vi "Clean Up.vi"(8 "error in (no error)":errorcluster, 11 "1553 Component in":refnum<class "1553 Component.lvclass">) -> (0 "error out":errorcluster)   [LabVIEW 2020, in "BCI-1553 API.lvlib" / "1553 Component.lvclass"]
doc: "Performs clean-up on the component. This will generally prepare the component in the 1553 Session to a known state and make it ready to accept a new configuration."
uses:
  1553 Component.lvclass
  1553 Component.lvclass/1553 Component.ctl
  Dependencies/FPGA Interface/FPGA Interface.lvclass
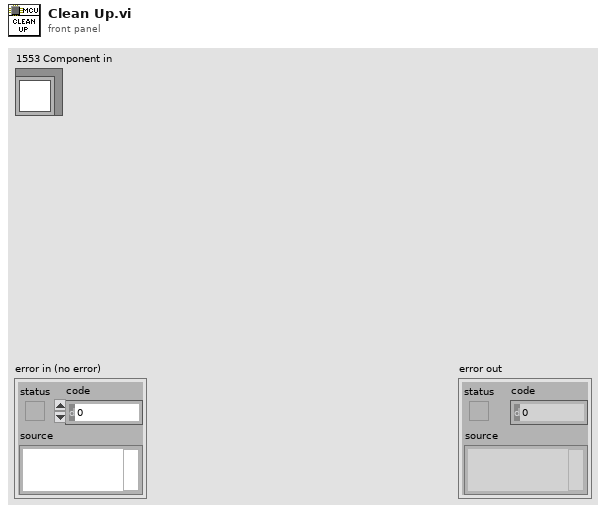
[diagram p1: front panel]
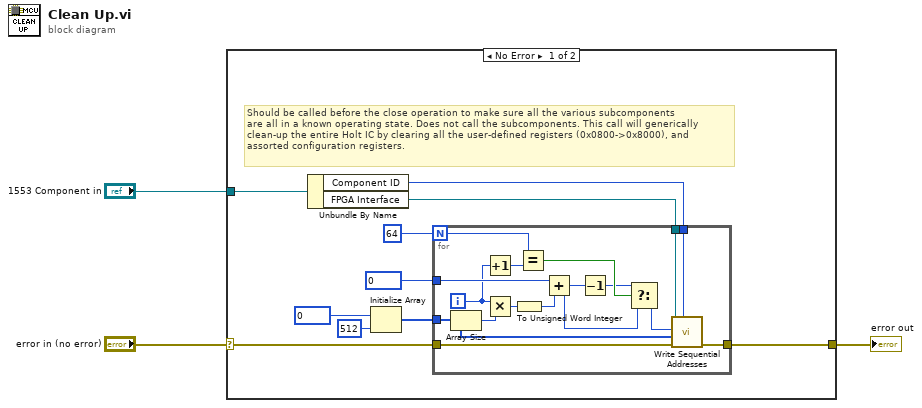
[diagram p0: block diagram]
diagram:
  n1 = case shown="No Error" "error in (no error)" {
    selector: "error in (no error)" -> [w10 w30]
    tunnel: [w9 w30] -> w2
    tunnel: "1553 Component in" -> [w13 _]
    frame No Error {
      # "Should be called before the close operation to make sure all the various subcomponents\nare all in a known operating state. Does not call the subcomponents. This call will generically\nclean-up the entire Holt IC by clearing all the user-defined registers (0x0800->0x8000), and\nassorted configuration registers."
      n2 = Unbundle By Name(w13) -> ("Component ID"=w11:u8, "FPGA Interface"=w12:refnum<class "FPGA Interface.lvclass">)
      n3 = Initialize Array(u16 0 ("Starting Address"), 512 ("dimension size")) -> (w5:u16[])
      n4 = for {
        N: 64 -> [w18]
        tunnel: w12 -> [w29]
        tunnel: w11 -> [w28]
        tunnel: u16 0 ("Starting Address") -> [w22]
        tunnel: w5 -> [w25]
        tunnel: w10 -> [w27]
        tunnel: [w26] -> w9
        i -> [w20]
        n5 = Array Size(array=w25) -> (size(s)=w24:i32)
        n6 = Increment(x=w20) -> (x+1=w19:i32)
        n7 = Multiply(x=w20, y=w24) -> (x*y=w23:i32)
        n8 = To Unsigned Word Integer(number=w23) -> (unsigned 16bit integer=w21:u16)
        n9 = Equal?(x=w18, y=w19) -> (x = y?=w17:bool)
        n10 = Add(x=w22, y=w21) -> (x+y=w15:u16)
        n11 = Decrement(x=w15) -> (x-1=w16:u16)
        n12 = Select(t=w16, s=w17, f=w15) -> (s? t:f=w14:u16)
        n13 = call-dynamic "Write Sequential Addresses.vi"("Target IC (1-8)"=w28, "error in (no error)"=w27, "Data"=w25, "Starting Address"=w14, "FPGA Interface in"=w29) -> ("error out"=w26:errorcluster)  [unwired: 6 in]
      }
    }
    frame Error {
    }
  }
  "error out" <- w2
